vi "SimpleDialog.vi"(10 "Data In":T1={"Btn"=FALSE, "Microprocessor"={"Port"="", "All Code"="Hi"}}, 11 "String in":refnum<vi>) -> ()   [LabVIEW 2016, in "BtnXControl.xctl"]
uses:
  BtnXControl.xctl
  uPythonX/uPythonX.xctl
  uPythonX/PythonData.ctl
  BtnData.ctl
panel:
  out "Console":string="\r\n>>> \r\nPYB: sync filesystems\r\nPYB: soft reboot\r\nMicroPython v1.10-210-g45076ee50-dirty on 2019-02-02; PYBD_SF2 with STM32F722IEK\r\nType \"help()\" for more information.\r\n>>> \r\n>>> import fwupdate\r\n>>> fwupdate.stage1()\r\nLoading file /flash/PYBD_SF2_W4F2_mboot.dfu.gz\r\nSupplied version of mboot is already on device.\r\nstage1 done, rebooting\r\nMicroPython v1.10-210-g45076ee50-dirty on 2019-02-02; PYBD_SF2 with STM32F722IEK\r\nType \"help()\" for more information.\r\n>>> \r\n>>> import fwupdate\r\n>>> fwupdate.stage2()\r\nstage2 done\r\n>>> \r\nPYB: sync filesystems\r\nPYB: soft reboot\r\nMicroPython v1.10-210-g45076ee50-dirty on 2019-02-02; PYBD_SF2 with STM32F722IEK\r\nType \"help()\" for more information.\r\n>>> \r\n>>> "
  in  "Test":bool
  in  "Cancel Button":bool
  in  "OK Button":bool
  in  "Settings":bool
  in  "Hub Port":u16(ring) items=["Red LED", "Green LED", "Motor A"]
  in  "USB Port":refnum<visa-resource-name>
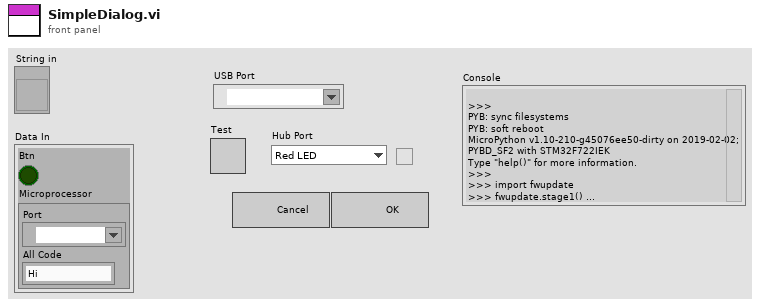
[diagram p1: front panel]
types:
  T1 = typedef "BtnXControl.xctl/BtnData.ctl" = cluster{"Btn":bool, "Microprocessor":T2}
  T2 = typedef "uPythonX.xctl/PythonData.ctl" = cluster{"Port":refnum<visa-resource-name>, "All Code":string}
  T3 = cluster{"USB Port":refnum<visa-resource-name>, string}
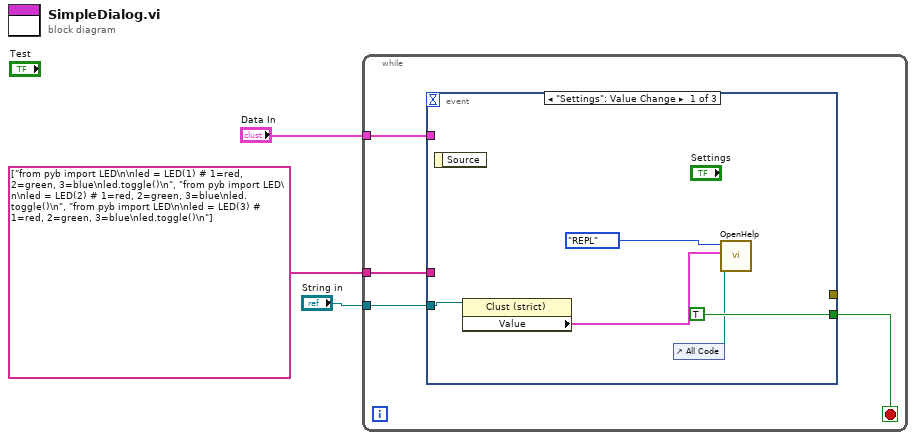
[diagram p0: block diagram]
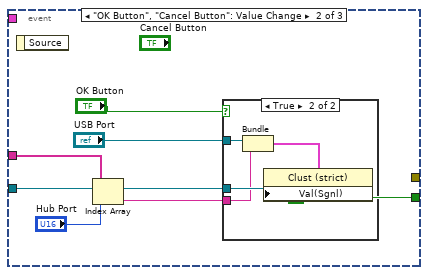
[diagram p2: hidden frame]
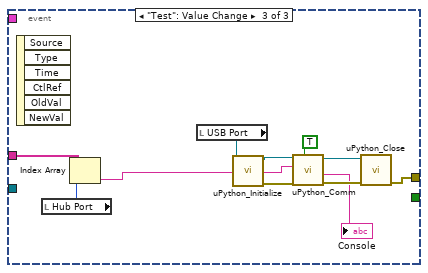
[diagram p4: hidden frame]
diagram:
  n1 = while {
    tunnel: "String in" -> [w7]
    tunnel: "Data In" -> [w6]
    tunnel: string[] ["from pyb import LED\n\nled = LED(1) # 1=red, 2=green, 3=blue\nled.toggle()\n", "from pyb import LED\n\nled = LED(2) # 1=red, 2=green, 3=blue\nled.toggle()\n", "from pyb import LED\n\nled = LED(3) # 1=red, 2=green, 3=blue\nled.toggle()\n"] -> [w4]
    stop <- w5 stop-if-true
    n2 = event shown="[0] \"Settings\": Value Change" {
      selector: _ -> [_ _ _]
      dyn-events: _ -> [_ _ _]
      timeout: _ -> [_ _ _]
      tunnel: w7 -> [w10 w15 _]
      tunnel: w6 -> [_ _ _]
      tunnel: [TRUE TRUE _] -> w5
      tunnel: w4 -> [_ w13 w27]
      tunnel: [_ _ w29] -> _
      event "Settings": Value Change {
        n3 = event-data() -> ()  [unwired: 1 in, 1 out]
        n4 = property class="Clust (strict)"(reference=w10) -> ("Value"=w9:T2)  [unwired: 1 in, 2 out]
        n5 = control-ref of="All Code"() -> (w8:refnum<vi>)
        n6 = call "OpenHelp.vi"("Code Ref"=w8, "Data In"=w9, "Dialog"=enum16{"REPL", "Help"}."REPL") -> ()  [unwired: 9 in]
      }
      event "OK Button", "Cancel Button": Value Change {
        n7 = event-data() -> ()  [unwired: 1 in, 1 out]
        n8 = Index Array(array=w13, index="Hub Port") -> (element=w16:string)
        n9 = case shown="True" "OK Button" {
          tunnel: w16 -> [_ w21]
          tunnel: w15 -> [_ w23]
          tunnel: "USB Port" -> [_ w22]
          frame False {
          }
          frame True {
            n10 = Bundle("USB Port"=w22, w21) -> (w20:T3)  [unwired: 1 in]
            n11 = property class="Clust (strict)"(reference=w23, "Val(Sgnl)"=w20) -> ()  [unwired: 1 in, 2 out]
          }
        }
      }
      event "Test": Value Change {
        n12 = event-data() -> ()  [unwired: 1 in, 6 out]
        n13 = local read "Hub Port"() -> (w26:u16)
        n14 = Index Array(array=w27, index=w26) -> (element=w25:string)
        n15 = local read "USB Port"() -> (w28:refnum<visa-resource-name>)
        n16 = call "uPython_Initialize.vi"("VISA Refnum in"=w28) -> ("error out"=w33:errorcluster, "VISA Refnum out"=w31:refnum<visa-resource-name>)  [unwired: 9 in]
        n17 = call "uPython_Comm.vi"("Wait for Reply?"=TRUE, "error in (no error)"=w33, "Script"=w25, "VISA Refnum in"=w31) -> ("error out"=w34:errorcluster, "Console Out"=→"Console":string, "VISA out"=w32:refnum<visa-resource-name>)  [unwired: 3 in, 2 out]
        n18 = call "uPython_Close.vi"("error in"=w34, "VISA  in"=w32) -> ("error out"=w29:errorcluster)  [unwired: 8 in, 1 out]
      }
    }
  }
